vi "Crosstalk Test.vi"(0 "VNA VISA":refnum<visa-resource-name>="TCPIP0::A-N5224A-41544.local::hislip0::INSTR", 1 "VNA Model:":enum16{"E5071C", "N5230A(C)", "N5224A"}(ring)=enum."N5224A", 2 "Channel":string="1", 4 "Demo Mode":bool, 5 "Sample PN:":string="1111111", 7 "SampleSN:":string="1111111", 9 "NEXT By Trace":bool) -> (14 "Fre":dbl[](array[numeric]), 15 "Data out":dbl[](array[numeric]), 17 "dup path":path)   [LabVIEW 2011]
panel:
  out "波形图":dbl[](graph)
  out "Find?":bool
  out "Points":i32
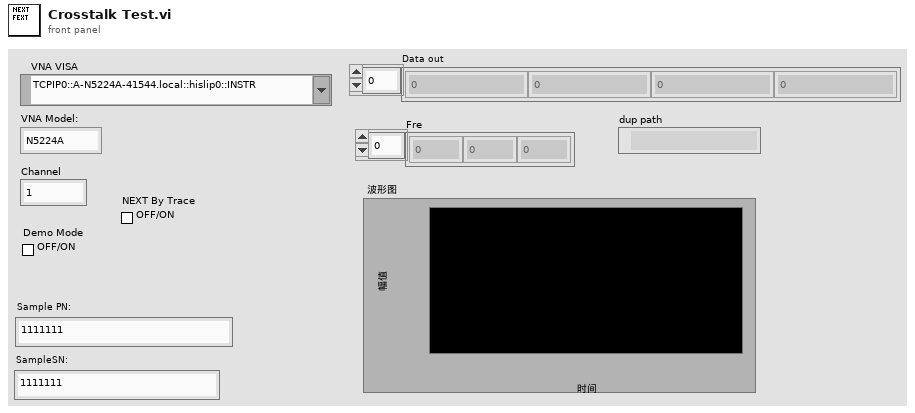
[diagram p1: front panel]
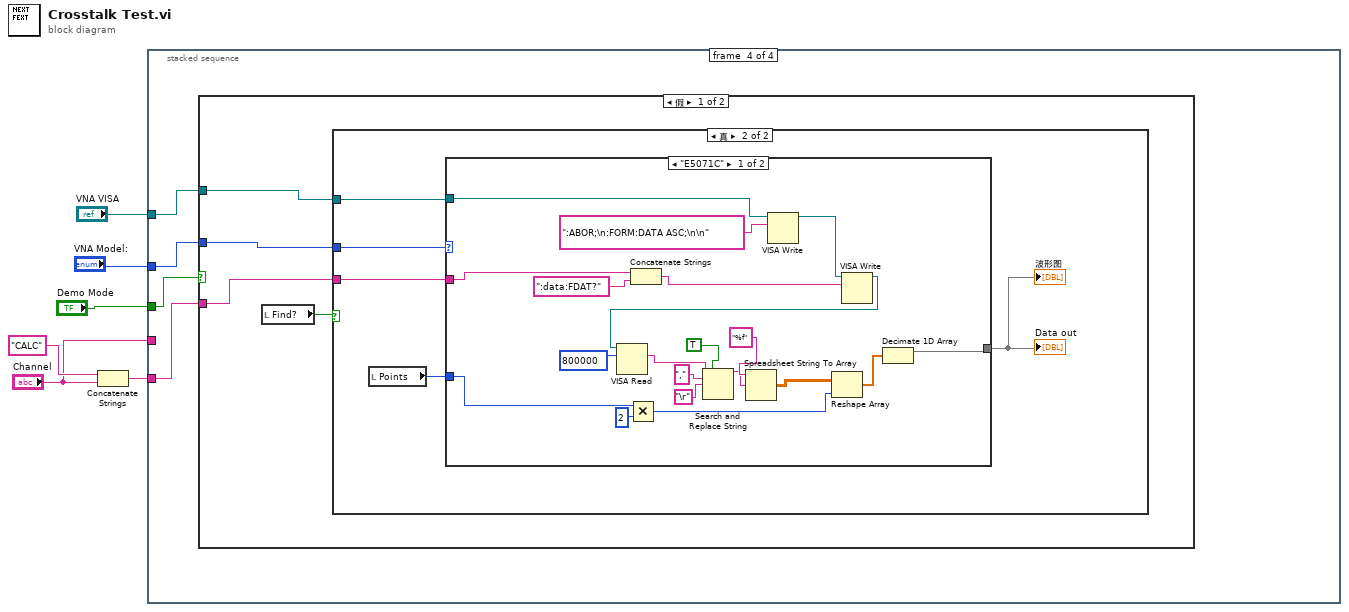
[diagram p0: block diagram]
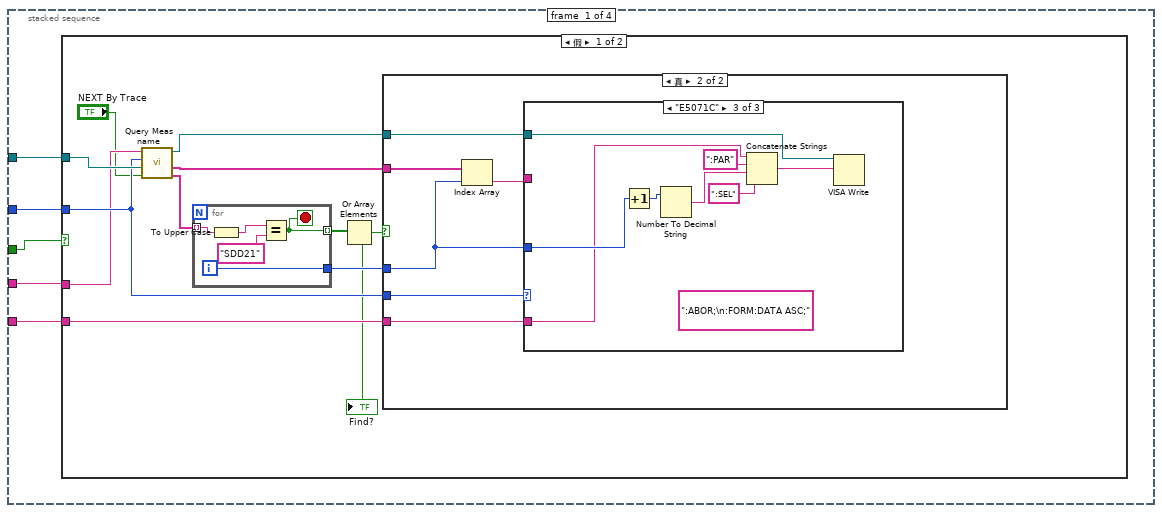
[diagram p2: hidden frame]
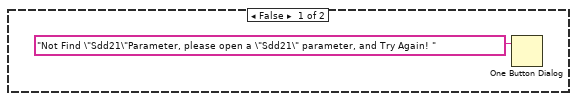
[diagram p3: hidden frame]
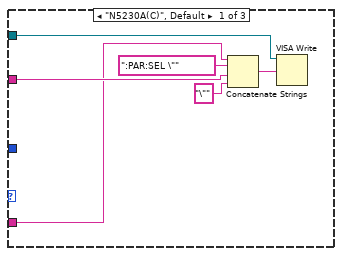
[diagram p4: hidden frame]
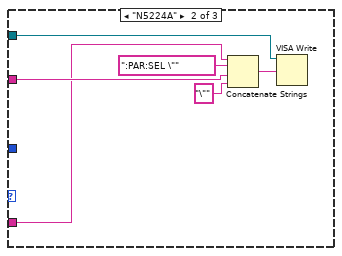
[diagram p5: hidden frame]
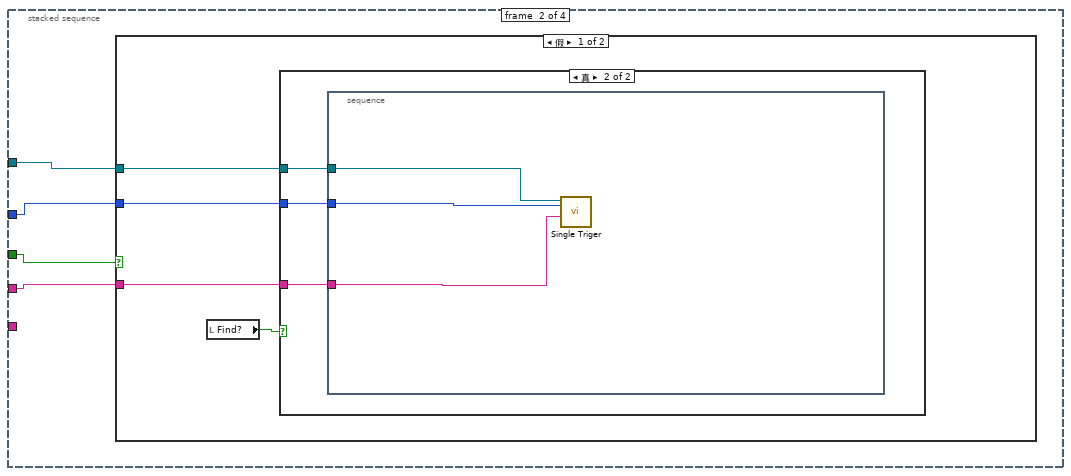
[diagram p7: hidden frame]
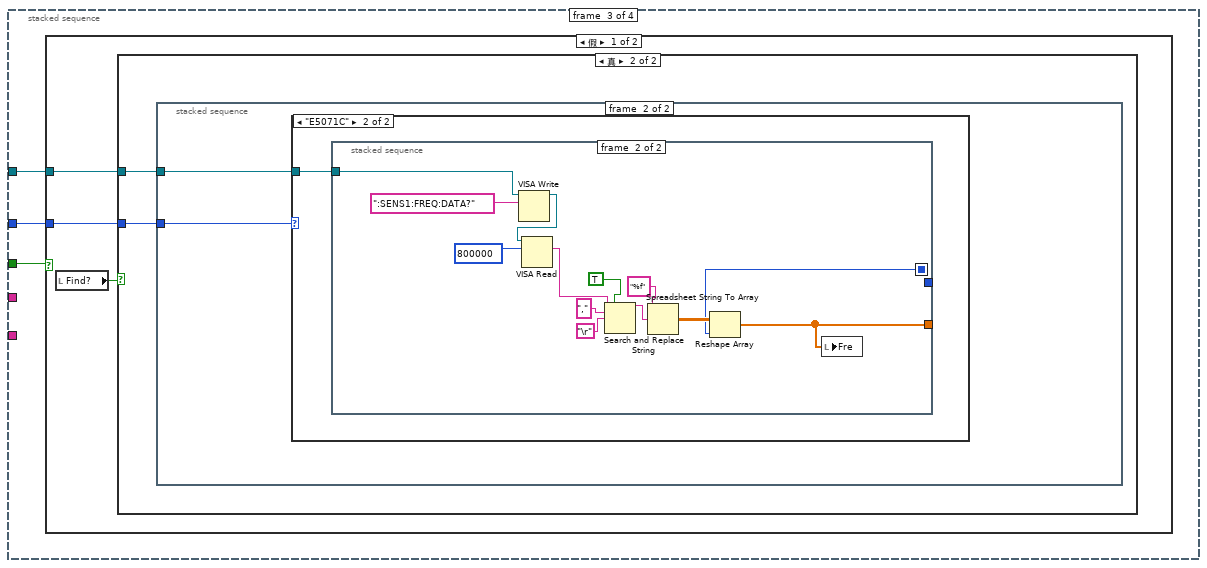
[diagram p10: hidden frame]
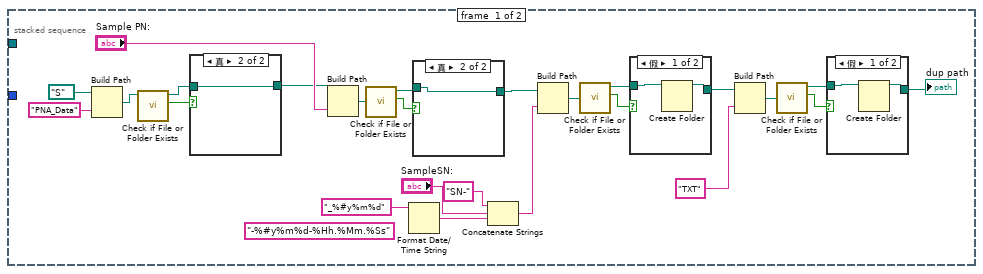
[diagram p12: hidden frame]
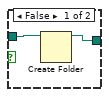
[diagram p15: hidden frame]
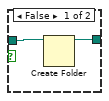
[diagram p16: hidden frame]
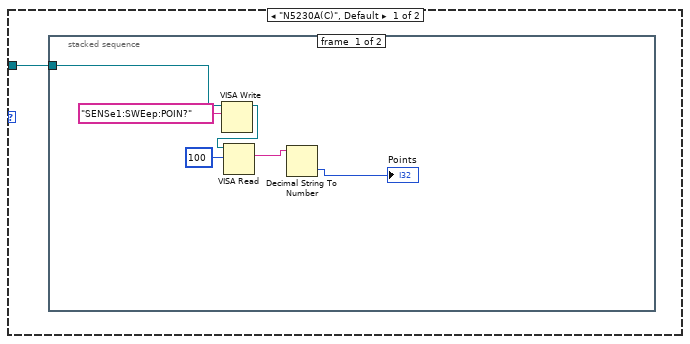
[diagram p17: hidden frame]
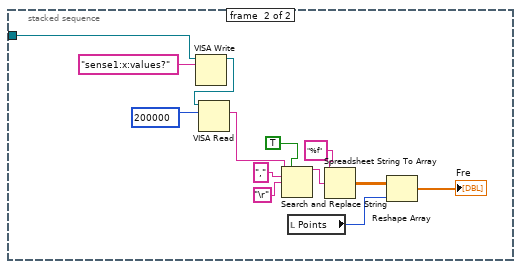
[diagram p18: hidden frame]
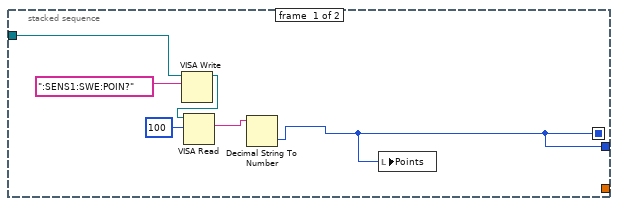
[diagram p19: hidden frame]
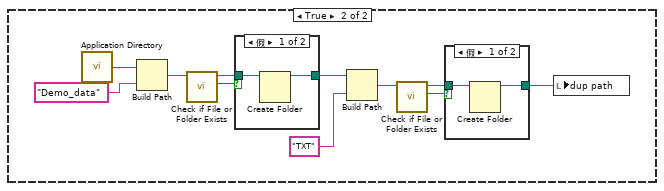
[diagram p20: hidden frame]
diagram:
  n1 = Concatenate Strings("CALC" ("字符串"), "Channel") -> (w2:string)
  n2 = stacked-sequence {
    tunnel: "VNA VISA" -> [w11 w58 w70 w176]
    tunnel: "VNA Model:" -> [w10 w57 w69 w175]
    tunnel: "Demo Mode" -> [w9 w56 w71 w174]
    tunnel: w2 -> [w7 _ _ w173]
    tunnel: "Channel" -> [w8 w55 _ _]
    frame #0 {
      n3 = case shown="假" w9 {
        tunnel: w11 -> [w22 _]
        tunnel: w10 -> [w19 _]
        tunnel: w8 -> [w18 _]
        tunnel: w7 -> [w17 _]
        frame False {
          n4 = call "Query Meas name.vi"("NEXT By Trace"="NEXT By Trace", "VISA resource name"=w22, "VNA Model"=w19, "Channel"=w18) -> ("Parameter item"=w16:string[], "Name list"=w21:string[], "Dup VISA resource name"=w20:refnum<visa-resource-name>)  [unwired: 3 in]
          n5 = for {
            tunnel: w16 -> [w51] mode=indexing
            tunnel: [w54] -> w14 mode=indexing
            tunnel: [w53] -> w15
            i -> [w53]
            stop <- w54 stop-if-true
            n6 = To Upper Case(1:w51) -> (0:w50:string)
            n7 = Equal?(x=w50, y="SDD21") -> (x = y?=w54:bool)
          }
          n8 = Or Array Elements(Boolean array=w14) -> (logical OR=w13:bool)
          "Find?" <- w13
          n9 = case shown="真" w13 {
            tunnel: w21 -> [_ w29]
            tunnel: w20 -> [_ w28]
            tunnel: w19 -> [_ w27]
            tunnel: w17 -> [_ w25]
            tunnel: w15 -> [_ w24]
            frame False {
              n10 = One Button Dialog(message="Not Find \"Sdd21\"Parameter, please open a \"Sdd21\" parameter, and Try Again! " ("消息")) -> ()  [unwired: 1 in, 1 out]
            }
            frame True {
              n11 = Index Array(array=w29, index=w24) -> (element=w26:string)
              n12 = case shown="\"E5071C\"" w27 {
                tunnel: w28 -> [w32 w38 w46]
                tunnel: w26 -> [w31 w37 _]
                tunnel: w24 -> [_ _ w44]
                tunnel: w25 -> [w30 w36 w42]
                frame "N5230A(C)", Default {
                  n13 = Concatenate Strings(w30, ":PAR:SEL \"", w31, "\"" ("string")) -> (w33:string)
                  n14 = VISA Write(VISA resource name=w32, write buffer=w33) -> ()  [unwired: 1 in, 3 out]
                }
                frame "N5224A" {
                  n15 = Concatenate Strings(w36, ":PAR:SEL \"", w37, "\"" ("string")) -> (w39:string)
                  n16 = VISA Write(VISA resource name=w38, write buffer=w39) -> ()  [unwired: 1 in, 3 out]
                }
                frame "E5071C" {
                  (unwired) ":ABOR;\n:FORM:DATA ASC;"
                  n17 = Increment(x=w44) -> (x+1=w45:i32)
                  n18 = Number To Decimal String(number=w45) -> (decimal integer string=w43:string)  [unwired: 1 in]
                  n19 = Concatenate Strings(w42, ":PAR" ("string"), w43, ":SEL" ("string")) -> (w49:string)
                  n20 = VISA Write(VISA resource name=w46, write buffer=w49) -> ()  [unwired: 1 in, 3 out]
                }
              }
            }
          }
        }
        frame True {
        }
      }
    }
    frame #1 {
      n21 = case shown="假" w56 {
        tunnel: w58 -> [w62 _]
        tunnel: w57 -> [w61 _]
        tunnel: w55 -> [w60 _]
        frame False {
          n22 = local read "Find?"() -> (w59:bool)
          n23 = case shown="真" w59 {
            tunnel: w62 -> [_ w65]
            tunnel: w61 -> [_ w64]
            tunnel: w60 -> [_ w63]
            frame False {
            }
            frame True {
              n24 = stacked-sequence {
                tunnel: w65 -> [w67]
                tunnel: w64 -> [w68]
                tunnel: w63 -> [w66]
                frame #0 {
                  n25 = call "Single Triger.vi"("Channel"=w66, "VNA Model:"=w68, "VISA"=w67) -> ()  [unwired: 9 in]
                }
              }
            }
          }
        }
        frame True {
        }
      }
    }
    frame #2 {
      n26 = case shown="假" w71 {
        tunnel: w70 -> [w74 _]
        tunnel: w69 -> [w73 _]
        frame False {
          n27 = local read "Find?"() -> (w72:bool)
          n28 = case shown="真" w72 {
            tunnel: w74 -> [_ w76]
            tunnel: w73 -> [_ w75]
            frame False {
            }
            frame True {
              n29 = stacked-sequence {
                tunnel: w75 -> [_ w115]
                tunnel: w76 -> [_ w114]
                frame #0 {
                  (unwired) "-%#y%m%d-%Hh.%Mm.%Ss" ("time format string (%c)")
                  n30 = Build Path(base path=path "S:/" ("基路径"), name or relative path="PNA_Data" ("名称或相对路径")) -> (appended path=w85:path)
                  n31 = call <vilib>:"Check if File or Folder Exists.vi"("path"=w85) -> ("file or folder exists?"=w86:bool, "dup path"=w87:path)  [unwired: 8 in, 1 out]
                  n32 = case shown="真" w86 {
                    tunnel: w87 -> [w112 w113]
                    tunnel: [w111 w113] -> w88
                    frame False {
                      n33 = Create Folder(path (use dialog)=w112) -> (created path=w111:path)  [unwired: 2 in, 2 out]
                    }
                    frame True {
                    }
                  }
                  n34 = Build Path(base path=w88, name or relative path="Sample PN:") -> (appended path=w90:path)
                  n35 = call <vilib>:"Check if File or Folder Exists.vi"("path"=w90) -> ("file or folder exists?"=w91:bool, "dup path"=w92:path)  [unwired: 8 in, 1 out]
                  n36 = Format Date/Time String(time format string (%c)="_%#y%m%d") -> (date/time string=w98:string)  [unwired: 2 in]
                  n37 = case shown="真" w91 {
                    tunnel: w92 -> [w109 w110]
                    tunnel: [w108 w110] -> w93
                    frame False {
                      n38 = Create Folder(path (use dialog)=w109) -> (created path=w108:path)  [unwired: 2 in, 2 out]
                    }
                    frame True {
                    }
                  }
                  n39 = Concatenate Strings("SN-" ("字符串"), "SampleSN:", w98) -> (w99:string)
                  n40 = Build Path(base path=w93, name or relative path=w99) -> (appended path=w94:path)
                  n41 = call <vilib>:"Check if File or Folder Exists.vi"("path"=w94) -> ("file or folder exists?"=w96:bool, "dup path"=w95:path)  [unwired: 8 in, 1 out]
                  n42 = case shown="假" w96 {
                    tunnel: w95 -> [w106 w107]
                    tunnel: [w105 w107] -> w78
                    frame False {
                      n43 = Create Folder(path (use dialog)=w106) -> (created path=w105:path)  [unwired: 2 in, 2 out]
                    }
                    frame True {
                    }
                  }
                  n44 = Build Path(base path=w78, name or relative path="TXT" ("名称或相对路径")) -> (appended path=w82:path)
                  n45 = call <vilib>:"Check if File or Folder Exists.vi"("path"=w82) -> ("file or folder exists?"=w80:bool, "dup path"=w81:path)  [unwired: 8 in, 1 out]
                  n46 = case shown="假" w80 {
                    tunnel: w81 -> [w103 w104]
                    tunnel: [w102 w104] -> w79
                    frame False {
                      n47 = Create Folder(path (use dialog)=w103) -> (created path=w102:path)  [unwired: 2 in, 2 out]
                    }
                    frame True {
                    }
                  }
                  "dup path" <- w79
                }
                frame #1 {
                  n48 = case shown="\"E5071C\"" w115 {
                    tunnel: w114 -> [w116 w136]
                    frame "N5230A(C)", Default {
                      n49 = stacked-sequence {
                        tunnel: w116 -> [w119 w125]
                        frame #0 {
                          n50 = VISA Write(VISA resource name=w119, write buffer="SENSe1:SWEep:POIN?") -> (VISA resource name out=w120:refnum<visa-resource-name>)  [unwired: 1 in, 2 out]
                          n51 = VISA Read(VISA resource name=w120, byte count=u32 100) -> (read buffer=w118:string)  [unwired: 1 in, 3 out]
                          n52 = Decimal String To Number(string=w118) -> (number=→"Points":i32)  [unwired: 2 in, 1 out]
                        }
                        frame #1 {
                          n53 = VISA Write(VISA resource name=w125, write buffer="sense1:x:values?") -> (VISA resource name out=w134:refnum<visa-resource-name>)  [unwired: 1 in, 2 out]
                          n54 = VISA Read(VISA resource name=w134, byte count=u32 200000) -> (read buffer=w133:string)  [unwired: 1 in, 3 out]
                          n55 = Search and Replace String(replace all?=TRUE ("replace all? (F)"), input string=w133, search string=",", replace string="\r") -> (result string=w129:string)  [unwired: 4 in, 3 out]
                          n56 = local read "Points"() -> (w123:i32)
                          n57 = Spreadsheet String To Array(format string="%f", spreadsheet string=w129) -> (array=w132:dbl[][])  [unwired: 2 in]
                          n58 = Reshape Array(w132, w123) -> (→"Fre":dbl[])
                        }
                      }
                    }
                    frame "E5071C" {
                      n59 = stacked-sequence {
                        seq-local: [w137 _] -> [_ w145]
                        tunnel: w136 -> [w140 w146]
                        tunnel: [_ w143] -> _
                        tunnel: [w137 _] -> _
                        frame #0 {
                          n60 = VISA Write(VISA resource name=w140, write buffer=":SENS1:SWE:POIN?") -> (VISA resource name out=w141:refnum<visa-resource-name>)  [unwired: 1 in, 2 out]
                          n61 = VISA Read(VISA resource name=w141, byte count=u32 100) -> (read buffer=w139:string)  [unwired: 1 in, 3 out]
                          n62 = Decimal String To Number(string=w139) -> (number=w137:i32)  [unwired: 2 in, 1 out]
                          n63 = local write "Points"(w137) -> ()
                        }
                        frame #1 {
                          n64 = VISA Write(VISA resource name=w146, write buffer=":SENS1:FREQ:DATA?") -> (VISA resource name out=w155:refnum<visa-resource-name>)  [unwired: 1 in, 2 out]
                          n65 = VISA Read(VISA resource name=w155, byte count=u32 800000) -> (read buffer=w154:string)  [unwired: 1 in, 3 out]
                          n66 = Search and Replace String(replace all?=TRUE ("replace all? (F)"), input string=w154, search string=",", replace string="\r") -> (result string=w150:string)  [unwired: 4 in, 3 out]
                          n67 = Spreadsheet String To Array(format string="%f", spreadsheet string=w150) -> (array=w153:dbl[][])  [unwired: 2 in]
                          n68 = Reshape Array(w153, w145) -> (w143:dbl[])
                          n69 = local write "Fre"(w143) -> ()
                        }
                      }
                    }
                  }
                }
              }
            }
          }
        }
        frame True {
          n70 = call <vilib>:"Application Directory.vi"() -> ("Application Directory"=w166:path)
          n71 = Build Path(base path=w166, name or relative path="Demo_data" ("名称或相对路径")) -> (appended path=w164:path)
          n72 = call <vilib>:"Check if File or Folder Exists.vi"("path"=w164) -> ("file or folder exists?"=w163:bool, "dup path"=w162:path)  [unwired: 8 in, 1 out]
          n73 = case shown="假" w163 {
            tunnel: w162 -> [w171 w172]
            tunnel: [w170 w172] -> w158
            frame False {
              n74 = Create Folder(path (use dialog)=w171) -> (created path=w170:path)  [unwired: 2 in, 2 out]
            }
            frame True {
            }
          }
          n75 = Build Path(base path=w158, name or relative path="TXT" ("名称或相对路径")) -> (appended path=w159:path)
          n76 = call <vilib>:"Check if File or Folder Exists.vi"("path"=w159) -> ("file or folder exists?"=w160:bool, "dup path"=w161:path)  [unwired: 8 in, 1 out]
          n77 = case shown="假" w160 {
            tunnel: w161 -> [w168 w169]
            tunnel: [w167 w169] -> w156
            frame False {
              n78 = Create Folder(path (use dialog)=w168) -> (created path=w167:path)  [unwired: 2 in, 2 out]
            }
            frame True {
            }
          }
          n79 = local write "dup path"(w156) -> ()
        }
      }
    }
    frame #3 {
      n80 = case shown="假" w174 {
        tunnel: w176 -> [w179 _]
        tunnel: w175 -> [w180 _]
        tunnel: w173 -> [w178 _]
        frame False {
          n81 = local read "Find?"() -> (w177:bool)
          n82 = case shown="真" w177 {
            tunnel: w180 -> [_ w185]
            tunnel: w179 -> [_ w184]
            tunnel: w178 -> [_ w183]
            frame False {
            }
            frame True {
              n83 = local read "Points"() -> (w182:i32)
              n84 = case shown="\"E5071C\"" w185 {
                tunnel: w184 -> [w189 w207]
                tunnel: [w205 w213] -> w181
                tunnel: w182 -> [w202 w212]
                tunnel: w183 -> [w188 w208]
                frame "E5071C" {
                  n85 = Multiply(x=w202, y=2) -> (x*y=w191:i32)
                  n86 = Concatenate Strings(w188, ":data:FDAT?" ("write buffer")) -> (w186:string)
                  n87 = VISA Write(VISA resource name=w189, write buffer=":ABOR;\n:FORM:DATA ASC;\n\n") -> (VISA resource name out=w203:refnum<visa-resource-name>)  [unwired: 1 in, 2 out]
                  n88 = VISA Write(VISA resource name=w203, write buffer=w186) -> (VISA resource name out=w193:refnum<visa-resource-name>)  [unwired: 1 in, 2 out]
                  n89 = VISA Read(VISA resource name=w193, byte count=u32 800000) -> (read buffer=w200:string)  [unwired: 1 in, 3 out]
                  n90 = Search and Replace String(replace all?=TRUE ("replace all? (F)"), input string=w200, search string=",", replace string="\r") -> (result string=w197:string)  [unwired: 4 in, 3 out]
                  n91 = Spreadsheet String To Array(format string="%f", spreadsheet string=w197) -> (array=w192:dbl[][])  [unwired: 2 in]
                  n92 = Reshape Array(w192, w191) -> (w190:dbl[])
                  n93 = Decimate 1D Array(w190) -> (w205:dbl[])  [unwired: 1 out]
                }
                frame "N5224A", Default {
                  n94 = Concatenate Strings(w208, ":DATA? FDATA" ("write buffer")) -> (w210:string)
                  n95 = VISA Write(VISA resource name=w207, write buffer=w210) -> (VISA resource name out=w215:refnum<visa-resource-name>)  [unwired: 1 in, 2 out]
                  n96 = VISA Read(VISA resource name=w215, byte count=u32 200000) -> (read buffer=w216:string)  [unwired: 1 in, 3 out]
                  n97 = Search and Replace String(replace all?=TRUE ("replace all? (F)"), input string=w216, search string=",", replace string="\r") -> (result string=w219:string)  [unwired: 4 in, 3 out]
                  n98 = Spreadsheet String To Array(format string="%f", spreadsheet string=w219) -> (array=w214:dbl[][])  [unwired: 2 in]
                  n99 = Reshape Array(w214, w212) -> (w213:dbl[])
                }
              }
              "Data out" <- w181
              "波形图" <- w181
            }
          }
        }
        frame True {
        }
      }
    }
  }
